vi "FTW-TransferClient-dotNET-Callback-ProgressUpload.vi"(4 "Initial Parameters":T1, 5 "Event Data":cluster{"sender":refnum<k24>, "e":refnum<k24>}, 6 "Control Ref":refnum<k24>, 7 "Event Common Data":T2) -> ()   [LabVIEW 2015, in "FTW-TransferClient-dotNET.lvclass"]
uses:
  FTW-TransferClient-dotNET.lvclass
  FTW-TransferClient-TransferProgress.ctl
  FTW-TransferClient.lvclass
panel:
  # "Inputs"
  # "Outputs"
  # "No Outputs - this VI\nis fire and forget"
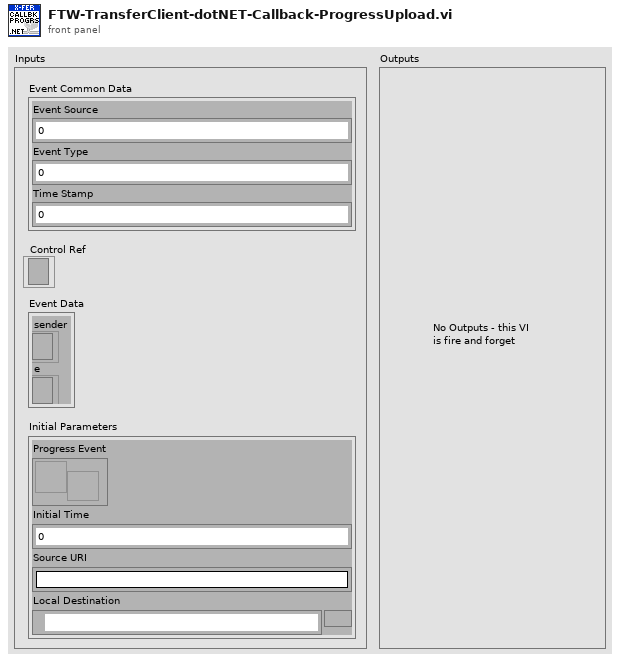
[diagram p1: front panel]
types:
  T1 = cluster{"Progress Event":refnum<user-event>, "Initial Time":u32, "Source URI":string, "Local Destination":path}
  T2 = cluster{"Event Source":i32, "Event Type":u32, "Time Stamp":u32}
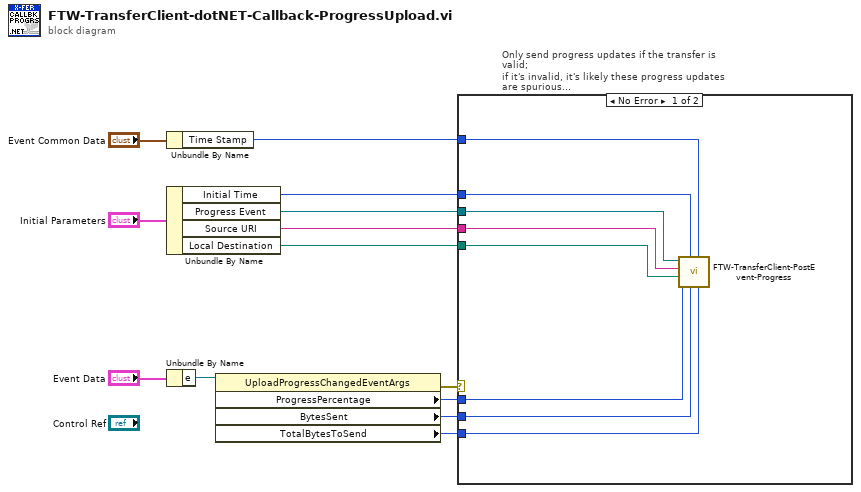
[diagram p0: block diagram]
diagram:
  n1 = Unbundle By Name("Event Common Data") -> ("Time Stamp"=w9:u32)
  n2 = Unbundle By Name("Initial Parameters") -> ("Initial Time"=w8:u32, "Progress Event"=w10:refnum<user-event>, "Source URI"=w7:string, "Local Destination"=w6:path)
  n3 = Unbundle By Name("Event Data") -> ("e"=w1:refnum<k24>)
  n4 = property class="UploadProgressChangedEventArgs"(reference=w1) -> (error out=w2:errorcluster, "ProgressPercentage"=w3:i32, "BytesSent"=w5:i64, "TotalBytesToSend"=w4:i64)  [unwired: 1 in, 1 out]
  n5 = case "Only send progress updates if the transfer is valid;\nif it's invalid, it's likely these progress updates are spurious\nattempts to contact the server (anecdotally;" shown="No Error" w2 {
    tunnel: w10 -> [w21 _]
    tunnel: w9 -> [w20 _]
    tunnel: w8 -> [w19 _]
    tunnel: w7 -> [w18 _]
    tunnel: w6 -> [w17 _]
    tunnel: w5 -> [w16 _]
    tunnel: w4 -> [w15 _]
    tunnel: w3 -> [w14 _]
    frame No Error {
      n6 = call "FTW-TransferClient-PostEvent-Progress.vi"("TotalBytes"=w15, "Timestamp"=w20, "TransferredBytes"=w16, "Initial Timestamp"=w19, "Percent Done"=w14, "Local Filepath"=w17, "Remote URI"=w18, "Transfer Progress Event"=w21) -> ()  [unwired: 4 in]
    }
    frame Error {
    }
  }
